vi "DepthSense NewFrame Callback With Globals.vi"(4 "User Parameter":variant, 6 "Control Ref":refnum<k24>, 7 "Event Common Data":T1) -> ()   [LabVIEW 2011]
uses:
  C:/Users/Behavior Room/Desktop/Kinect Mouse/DepthSense/FunctionPointerProxy/FunctionPointerProxy/bin/Release/FunctionPointerProxy.dll
  FunctionPointerProxy/FunctionPointerProxy/bin/Release/FunctionPointerProxy.dll
  DepthSense Global Status.vi
  <userlib>/libOptrima-2-3/libOptrima-2-3.lvlib
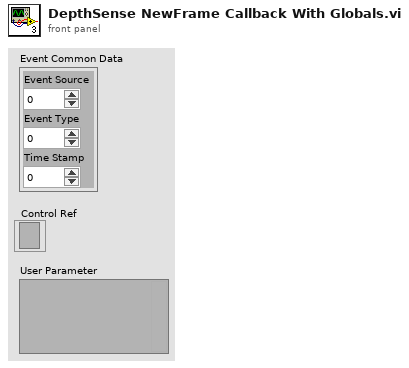
[diagram p1: front panel]
types:
  T1 = cluster{"Event Source":i32, "Event Type":u32, "Time Stamp":u32}
  T2 = typedef "DepthSense State.ctl" = cluster{"Camera Version":string, "Image Height":i32, "Image Width":i32, "Minimum Framerate":i32, "Maximum Framerate":i32, "Framerate":i32, "Close Mode":bool, "Denoising":bool, "Leakage Algorithm":bool, "Anti-Aliasing":bool, "Camera Status":i32, "API Version":string, "Light Intensity":i32}
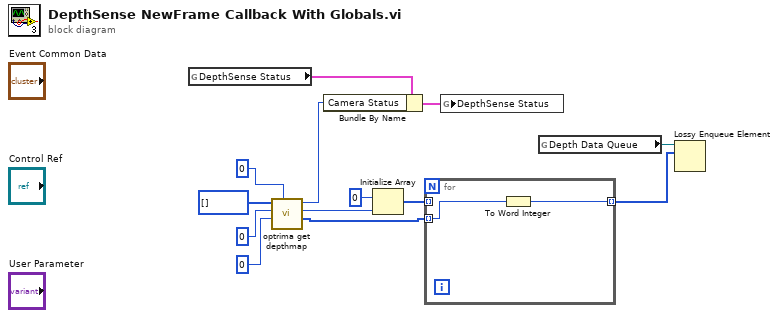
[diagram p0: block diagram]
diagram:
  n1 = global read "DepthSense Global Status.vi" "DepthSense Status"() -> (w7:T2)
  n2 = call <userlib>:"optrima get depthmap.vi"("to_camera_plane"=0, "confidenceTH"=i16 0 ("confidence_threshold"), "length"=u32 0, "p_depthmap in"=u16[] []) -> ("p_depthmap out"=w2:u16[], "length out"=w9:u32, "function return"=w6:u32)  [unwired: 4 in, 1 out]
  n3 = Bundle By Name(cluster=w7, "Camera Status"=w6) -> (w5:T2)
  n4 = Initialize Array(i16 0 ("element"), w9) -> (w3:i16[])
  n5 = for {
    tunnel: w3 -> [_] mode=indexing
    tunnel: w2 -> [w15] mode=indexing
    tunnel: [w14] -> w1 mode=indexing
    n6 = To Word Integer(number=w15) -> (16bit integer=w14:i16)
  }
  n7 = global write "DepthSense Global Status.vi" "DepthSense Status"(w5) -> ()
  n8 = global read "DepthSense Global Status.vi" "Depth Data Queue"() -> (w8:refnum<queue>)
  n9 = Lossy Enqueue Element(queue=w8, element=w1) -> ()  [unwired: 1 in, 4 out]
